vi "Test1 - Measure Frequency.vi"(11 "IO":T1) -> (3 "Node":refnum<class "bt_Node.lvclass">)   [LabVIEW 2021, in "Test Sequencer Support.lvlib"]
uses:
  Test Sequencer Support.lvlib
  IO Type.ctl
  <vilib>/TSA/Event Log/Event_TextLog/Event_TextLog.lvclass
  C:/Program Files (x86)/National Instruments/LabVIEW 2021/vi.lib/TSA/Event Log/abs_EventLog/abs_EventLog.lvclass
  Blackboard/Blackboard.lvclass
  <vilib>/TSA/Abstract Data Classes/Abs_Types/Boolean/Abs_Boolean.lvclass
  C:/Program Files (x86)/National Instruments/LabVIEW 2021/vi.lib/TSA/Abstract Data Classes/Abs_Types/Type/Abs_Type.lvclass
  <vilib>/TSA/Abstract Data Classes/Abs_Types/Waveform/Abs_Waveform.lvclass
  <vilib>/TSA/Abstract Data Classes/Abs_Types/Double Float/Abs_Double Float.lvclass
  Support/Nodes/abs_Node/bt_Node.lvclass
  Support/Nodes/Leaves/abs_Type Leaf/abs_Type Leaf.lvclass/abs_Type Leaf.ctl
  Support/Nodes/Leaves/abs_Type Leaf/Properties/Write Value Class.vi
  <vilib>/TSA/Abstract Data Classes/Constants/Support/DBL/Const_DBL.lvclass
  C:/Program Files (x86)/National Instruments/LabVIEW 2021/vi.lib/TSA/Abstract Data Classes/Abs_Types/Numeric/Abs_Numeric.lvclass
  Support/Nodes/Leaves/Log/bt_Log.lvclass
  C:/Users/timst/Documents/Repositories/LV_Behaviour_Tree/Source/Support/Nodes/abs_Node/bt_Node.lvclass
  Support/Nodes/Leaves/Test Boolean/Test Abs_Boolean.lvclass
  C:/Users/timst/Documents/Repositories/LV_Behaviour_Tree/Source/Support/Nodes/Leaves/abs_Type Leaf/abs_Type Leaf.lvclass
  Nodes/Measure Waveform/Measure Waveform.lvclass
  Support/Poly/Log/Log_StringClass.vi
  <vilib>/TSA/Abstract Data Classes/Constants/Support/DBL/DBL.vi
  <vilib>/TSA/Abstract Data Classes/Functions/Compare/Support/Greater Equal/DBL/Method.vi
  <vilib>/TSA/Abstract Data Classes/Functions/Compare/Support/Less Equal/DBL/Method.vi
  <vilib>/TSA/Abstract Data Classes/Functions/Logic/Support/AND/Bool/Method.vi
  BT.lvlib
  C:/Program Files (x86)/National Instruments/LabVIEW 2021/vi.lib/TSA/Abstract Data Classes/Abs_Types/Double Float/Abs_Double Float.lvclass
  C:/Program Files (x86)/National Instruments/LabVIEW 2021/vi.lib/TSA/Abstract Data Classes/Abs_Types/Floating Point/Abs_Floating Point.lvclass
  C:/Program Files (x86)/National Instruments/LabVIEW 2021/vi.lib/TSA/Abstract Data Classes/Abs_Types/Value/Abs_Value.lvclass
  C:/Program Files (x86)/National Instruments/LabVIEW 2021/vi.lib/TSA/Abstract Data Classes/Constants/Support/DBL/Const_DBL.lvclass
  C:/Program Files (x86)/National Instruments/LabVIEW 2021/vi.lib/TSA/Abstract Data Classes/Constants/Support/Interface/Const_Intf.lvclass
  <vilib>/TSA/Abstract Data Classes/Functions/Compare/Support/Greater Equal/DBL/Greater Equal_DBL.lvclass
  <vilib>/TSA/Abstract Data Classes/Functions/Logic/Support/AND/Bool/AND_Bool.lvclass
  <vilib>/TSA/Abstract Data Classes/Functions/Compare/Support/Less Equal/DBL/Less Equal_DBL.lvclass
  C:/Program Files (x86)/National Instruments/LabVIEW 2021/vi.lib/TSA/Event Log/Event_TextLog/Event_TextLog.lvclass
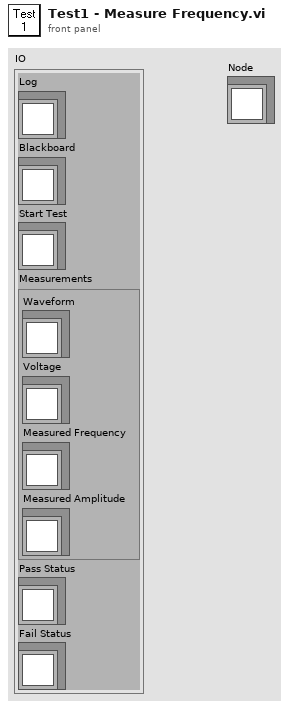
[diagram p1: front panel]
types:
  T1 = typedef "Test Sequencer Support.lvlib/IO Type.ctl" = cluster{"Log":refnum<class "Event_TextLog.lvclass">, "Blackboard":refnum<class "Blackboard.lvclass">, "Start Test":refnum<class "Abs_Boolean.lvclass">, "Measurements":cluster{"Waveform":refnum<class "Abs_Waveform.lvclass">, "Voltage":refnum<class "Abs_Double Float.lvclass">, "Measured Frequency":refnum<class "Abs_Double Float.lvclass">, "Measured Amplitude":refnum<class "Abs_Double Float.lvclass">}, "Pass Status":refnum<class "Abs_Boolean.lvclass">, "Fail Status":refnum<class "Abs_Boolean.lvclass">}
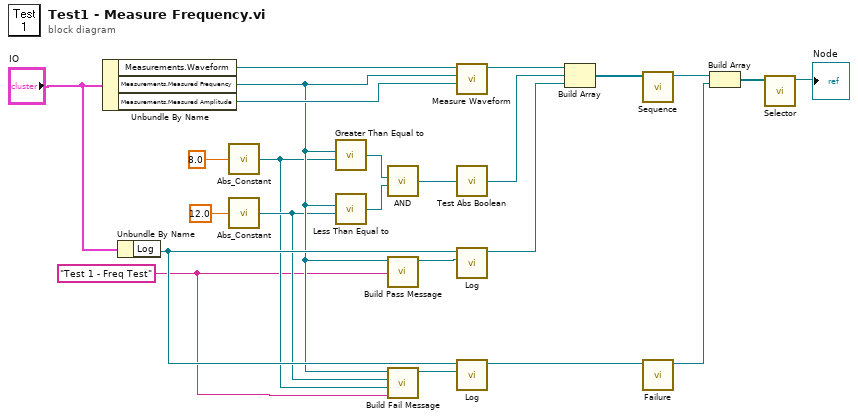
[diagram p0: block diagram]
diagram:
  w1 = "Test 1 - Freq Test" ("Name")
  n1 = Unbundle By Name("IO") -> ("Measurements.Waveform"=w24:refnum<class "Abs_Waveform.lvclass">, "Measurements.Measured Frequency"=w4:refnum<class "Abs_Double Float.lvclass">, "Measurements.Measured Amplitude"=w23:refnum<class "Abs_Double Float.lvclass">)
  n2 = Unbundle By Name("IO") -> ("Log"=w7:refnum<class "Event_TextLog.lvclass">)
  n3 = call-poly <vilib>:"Abs_Constant.vi"("Value"=8.0 ("Lower Limit")) -> ("Constant"=w2:refnum<class "Const_DBL.lvclass">)  [unwired: 4 in]
  n4 = call-poly <vilib>:"Abs_Constant.vi"("Value"=12.0 ("Upper Limit")) -> ("Constant"=w3:refnum<class "Const_DBL.lvclass">)  [unwired: 4 in]
  n5 = call-poly <vilib>:"Greater Than Equal to.vi"("Value B"=w2, "Value A"=w4) -> ("Result"=w20:refnum<class "Abs_Boolean.lvclass">)  [unwired: 4 in]
  n6 = call-poly <vilib>:"Less Than Equal to.vi"("Value B"=w3, "Value A"=w4) -> ("Result"=w19:refnum<class "Abs_Boolean.lvclass">)  [unwired: 4 in]
  n7 = call-poly <vilib>:"AND.vi"("B"=w19, "A"=w20) -> ("Result"=w18:refnum<class "Abs_Boolean.lvclass">)  [unwired: 4 in]
  n8 = call "Build Pass Message.vi"("Test Name"=w1, "Result"=w4) -> ("Abs_String out"=w6:refnum<class "Abs_String.lvclass">)  [unwired: 9 in]
  n9 = call "Build Fail Message.vi"("Test Name"=w1, "Lower Limit"=w2, "Upper Limit"=w3, "Result"=w4) -> ("Abs_String out"=w5:refnum<class "Abs_String.lvclass">)  [unwired: 7 in]
  n10 = call "Measure Waveform.vi"("Measured Amplitude"=w23, "Measured Frequency"=w4, "Abs_Waveform in"=w24) -> ("Measure Waveform out"=w22:refnum<class "Measure Waveform.lvclass">)  [unwired: 8 in]
  n11 = call "Test Abs Boolean.vi"("Abs_Boolean.lvclass"=w18) -> ("abs_Node"=w17:refnum<class "bt_Node.lvclass">)  [unwired: 4 in]
  n12 = call-poly "Log.vi"("Message"=w6, "EventLog"=w7) -> ("node out"=w13:refnum<class "bt_Log.lvclass">)  [unwired: 9 in]
  n13 = call-poly "Log.vi"("Message"=w5, "EventLog"=w7) -> ("node out"=w11:refnum<class "bt_Log.lvclass">)  [unwired: 9 in]
  n14 = Build Array(w22, w17, w13) -> (w21:refnum<class "bt_Node.lvclass">[])
  n15 = call "Sequence.vi"("Nodes"=w21) -> ("Node"=w15:refnum<class "bt_Node.lvclass">)  [unwired: 10 in]
  n16 = call "Failure.vi"("Node In"=w11) -> ("Node"=w12:refnum<class "bt_Node.lvclass">)  [unwired: 10 in]
  n17 = Build Array(w15, w12) -> (w14:refnum<class "bt_Node.lvclass">[])
  n18 = call "Selector.vi"("Nodes"=w14) -> ("Node"=→"Node":refnum<class "bt_Node.lvclass">)  [unwired: 10 in]
